vi "Color Picker Dialog (.NET).vi"(8 "error in (no error)":errorcluster, 10 "VI Reference":refnum<vi>, 11 "Color in":u32(colorbox)=16711680) -> (0 "error out":errorcluster, 1 "Cancelled":bool, 3 "Color out":u32(colorbox))   [LabVIEW 2015]
uses:
  System.Drawing
  System.Windows.Forms
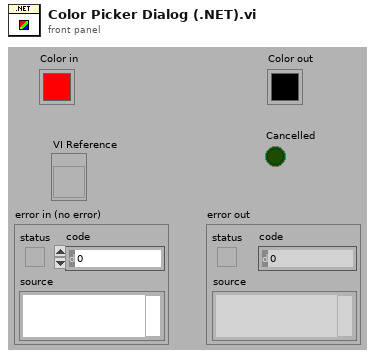
[diagram p1: front panel]
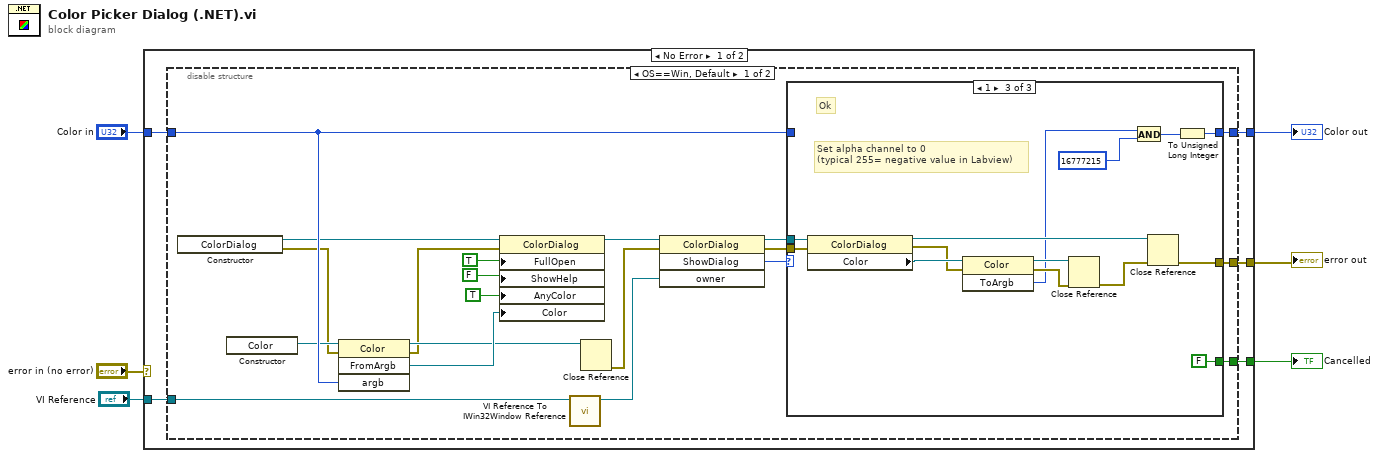
[diagram p0: block diagram]
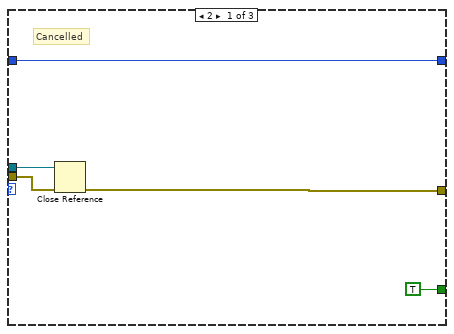
[diagram p2: hidden frame]
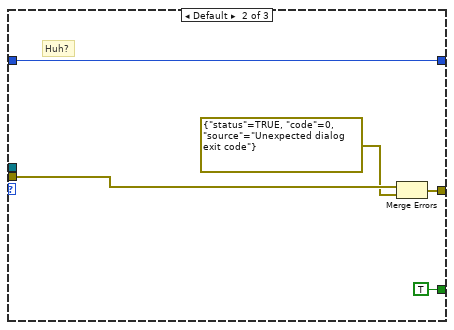
[diagram p3: hidden frame]
diagram:
  n1 = case shown="No Error" "error in (no error)" {
    selector: "error in (no error)" -> [_ w57]
    tunnel: [w9 w57] -> w6
    tunnel: "Color in" -> [w10 _]
    tunnel: [w11 _] -> w3
    tunnel: [w7 _] -> w2
    tunnel: "VI Reference" -> [w8 _]
    frame No Error {
      n2 = disable-structure shown="OS==Win, Default" {
        disable-tunnel: [w31 w56] -> w11
        disable-tunnel: w10 -> [w30 w56]
        disable-tunnel: [w29 _] -> w9
        disable-tunnel: w8 -> [w28 _]
        disable-tunnel: [w27 _] -> w7
        frame condition #0 (active) {
          n3 = constructor class="ColorDialog"() -> (reference out=w22:refnum<k24>, error out=w15:errorcluster)  [unwired: 3 in, 1 out]
          n4 = constructor class="Color"() -> (reference out=w19:refnum<k24>)  [unwired: 3 in, 2 out]
          n5 = invoke class="Color" method="FromArgb"(reference=w19, error in=w15, "argb"=w30) -> (reference out=w17:refnum<k24>, error out=w14:errorcluster, "FromArgb"=w18:refnum<k24>)  [unwired: 1 in, 1 out]
          n6 = property class="ColorDialog"(reference=w22, error in=w14, "FullOpen"=TRUE, "ShowHelp"=FALSE ("AnyColor"), "AnyColor"=TRUE, "Color"=w18) -> (reference out=w23:refnum<k24>)  [unwired: 1 out]
          n7 = call "VI Reference To IWin32Window Reference.vi"("VI Reference"=w28) -> ("System.Windows.Forms.IWin32Window"=w12:refnum<k24>)  [unwired: 9 in, 1 out]
          n8 = Close Reference(reference=w17) -> (error out=w16:errorcluster)  [unwired: 1 in]
          n9 = invoke class="ColorDialog" method="ShowDialog"(reference=w23, error in=w16, "owner"=w12) -> (reference out=w21:refnum<k24>, error out=w13:errorcluster, "ShowDialog"=w20:i32)  [unwired: 1 in, 1 out]
          n10 = case shown="1" w20 {
            tunnel: w21 -> [w35 _ w55]
            tunnel: w13 -> [w34 w40 w54]
            tunnel: w30 -> [w36 w41 _]
            tunnel: [w36 w41 w47] -> w31
            tunnel: [w33 w38 w43] -> w29
            tunnel: [TRUE TRUE FALSE] -> w27
            frame 2 {
              (unwired) TRUE
              # "Cancelled"
              n11 = Close Reference(reference=w35, error in (no error)=w34) -> (error out=w33:errorcluster)
            }
            frame Default {
              # "Huh?"
              n12 = Merge Errors(w40, errorcluster {"status"=TRUE, "code"=0, "source"="Unexpected dialog exit code"} ("error in 2 (no error)")) -> (w38:errorcluster)
            }
            frame 1 {
              # "Set alpha channel to 0\n(typical 255= negative value in Labview)"
              # "Ok"
              n13 = property class="ColorDialog"(reference=w55, error in=w54) -> (reference out=w53:refnum<k24>, error out=w49:errorcluster, "Color"=w51:refnum<k24>)
              n14 = invoke class="Color" method="ToArgb"(reference=w51, error in=w49) -> (reference out=w50:refnum<k24>, error out=w48:errorcluster, "ToArgb"=w46:i32)  [unwired: 1 in]
              n15 = Close Reference(reference=w50, error in (no error)=w48) -> (error out=w52:errorcluster)
              n16 = And(x=w46, y=16777215) -> (x .and. y?=w44:i32)
              n17 = Close Reference(reference=w53, error in (no error)=w52) -> (error out=w43:errorcluster)
              n18 = To Unsigned Long Integer(number=w44) -> (unsigned 32bit integer=w47:u32)
            }
          }
        }
        frame condition #1 {
        }
      }
    }
    frame Error {
    }
  }
  "error out" <- w6
  "Color out" <- w3
  "Cancelled" <- w2
